vi "color image 2d.vi"(6 "path to JPEG file":path, 7 "Max":i32, 8 "Names":T2={"Red name"="Ca", "Green name"="Ca", "Blu name"="Ca"}, 9 "ROI-Blue":i32[][](graph), 10 "ROI-Green":i32[][](graph), 11 "ROI-Red":i32[][](graph)) -> ()   [LabVIEW 2023]
uses:
  <vilib>/Utility/miscctls.llb/LVBoundsTypeDef.ctl
  <vilib>/vision/Management.llb/Cast Image 2 Method.ctl
  <vilib>/vision/NI_Vision_Development_Module.lvlib
panel:
  out "Red":T1(plugin-control)
  out "Green":T1(plugin-control)
  out "Blue":T1(plugin-control)
  out "concatenated string":picture
  out "error out":errorcluster
  in  "error in":errorcluster
  out "Intensity Graph 6":u16[][](graph)
  out "Intensity Graph 5":u16[][](graph)
  out "Intensity Graph 4":u16[][](graph)
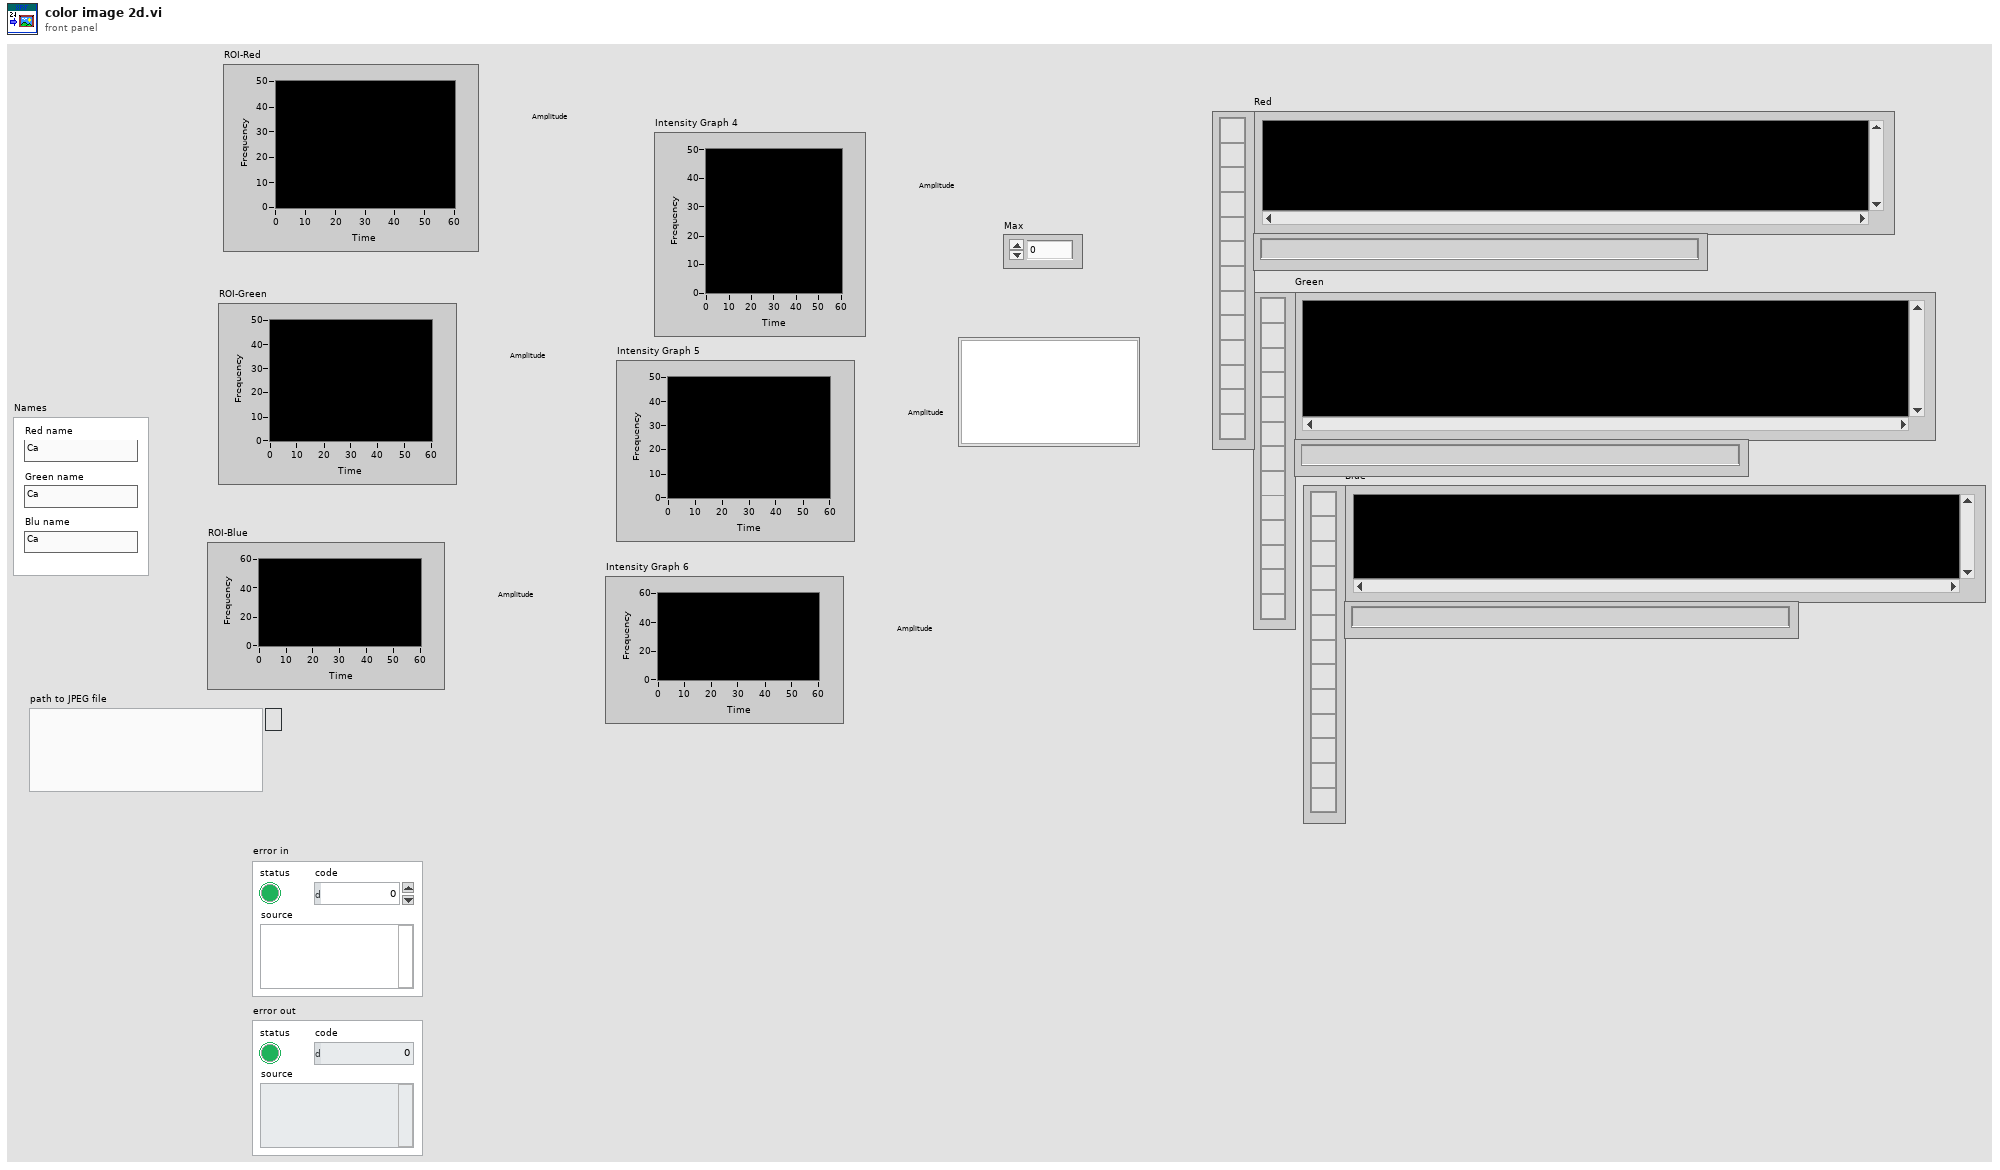
[diagram p1: front panel]
types:
  T1 = typedef "IMAQ Image.ctl" = refnum<image>
  T2 = cluster{"Red name":string, "Green name":string, "Blu name":string}
  T3 = typedef "Image Type" = u32
  T4 = typedef "Cast Image 2 Method.ctl" = u32
  T5 = typedef "LVBoundsTypeDef.ctl" = cluster{"Width":u32, "Height":u32}
  T6 = enum16{"User-specified Font", "Application Font", "System Font", "Dialog Font"}
  T7 = cluster{"Font Name:":string, "Size":i16, "Strikeout?":bool, "Italic?":bool, "Underline?":bool, "Outline?":bool, "Shadow?":bool, "Bold?":bool}
  T8 = typedef "imagedata.ctl" = cluster{"image type":i32, "image depth":i32, "image":u8[], "mask":u8[], "colors":u32[], "Rectangle":cluster{"left":i16, "top":i16, "right":i16, "bottom":i16}}
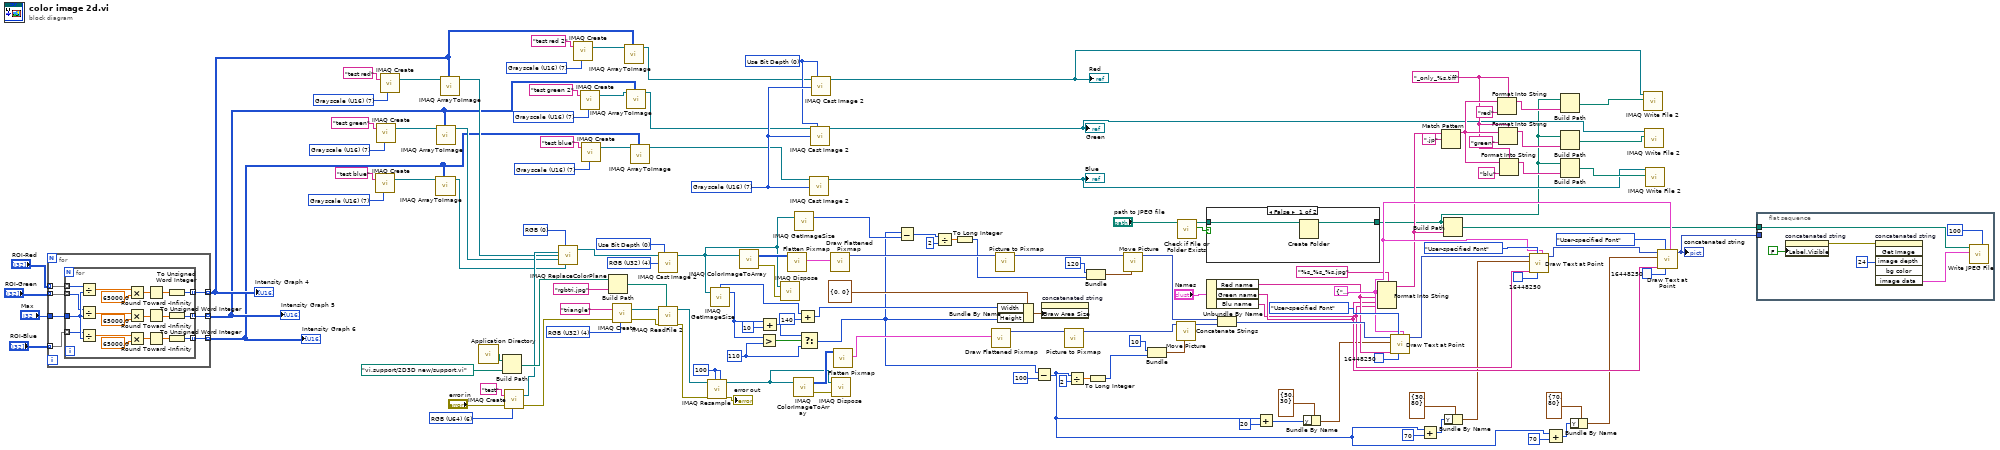
[diagram p0: block diagram]
diagram:
  w11 = T3 7 items=["Grayscale (U8)", "Grayscale (I16)", "Grayscale (SGL)", "Complex (CSG)", "RGB (U32)", "HSL (U32)", "RGB (U64)", "Grayscale (U16)"] ("Image Type")
  w13 = T3 7 items=["Grayscale (U8)", "Grayscale (I16)", "Grayscale (SGL)", "Complex (CSG)", "RGB (U32)", "HSL (U32)", "RGB (U64)", "Grayscale (U16)"] ("Image Type")
  w14 = T3 7 items=["Grayscale (U8)", "Grayscale (I16)", "Grayscale (SGL)", "Complex (CSG)", "RGB (U32)", "HSL (U32)", "RGB (U64)", "Grayscale (U16)"] ("Image Type")
  w17 = T4 0 items=["Use Bit Depth", "Shift", "Use Lookup Table"] ("Method")
  w18 = T3 7 items=["Grayscale (U8)", "Grayscale (I16)", "Grayscale (SGL)", "Complex (CSG)", "RGB (U32)", "HSL (U32)", "RGB (U64)", "Grayscale (U16)"] ("Image Type")
  w35 = "_only_%s.tiff" ("format string")
  w70 = u16 0 items=["RGB", "HSL", "HSV", "HSI"] ("Color Mode")
  w79 = T3 7 items=["Grayscale (U8)", "Grayscale (I16)", "Grayscale (SGL)", "Complex (CSG)", "RGB (U32)", "HSL (U32)", "RGB (U64)", "Grayscale (U16)"] ("Image Type")
  w76 = T3 7 items=["Grayscale (U8)", "Grayscale (I16)", "Grayscale (SGL)", "Complex (CSG)", "RGB (U32)", "HSL (U32)", "RGB (U64)", "Grayscale (U16)"] ("Image Type")
  w73 = T3 7 items=["Grayscale (U8)", "Grayscale (I16)", "Grayscale (SGL)", "Complex (CSG)", "RGB (U32)", "HSL (U32)", "RGB (U64)", "Grayscale (U16)"] ("Image Type")
  w84 = T3 4 items=["Grayscale (U8)", "Grayscale (I16)", "Grayscale (SGL)", "Complex (CSG)", "RGB (U32)", "HSL (U32)", "RGB (U64)", "Grayscale (U16)"] ("Image Type")
  w85 = T4 0 items=["Use Bit Depth", "Shift", "Use Lookup Table"] ("Method")
  w64 = u32 110 ("Height")
  w101 = T7 {"Font Name:"="Times", "Size"=18, "Strikeout?"=FALSE, "Italic?"=FALSE, "Underline?"=FALSE, "Outline?"=FALSE, "Shadow?"=FALSE, "Bold?"=TRUE} ("[user-specified font]")
  w125 = T3 4 items=["Grayscale (U8)", "Grayscale (I16)", "Grayscale (SGL)", "Complex (CSG)", "RGB (U32)", "HSL (U32)", "RGB (U64)", "Grayscale (U16)"] ("Image Type")
  w129 = 100
  w138 = T3 6 items=["Grayscale (U8)", "Grayscale (I16)", "Grayscale (SGL)", "Complex (CSG)", "RGB (U32)", "HSL (U32)", "RGB (U64)", "Grayscale (U16)"] ("Image Type")
  n1 = for {
    tunnel: "ROI-Red" -> [w150] mode=indexing
    tunnel: "ROI-Green" -> [w149] mode=indexing
    tunnel: "ROI-Blue" -> [w148] mode=indexing
    tunnel: "Max" -> [w147]
    tunnel: [w146] -> w6 mode=indexing
    tunnel: [w145] -> w5 mode=indexing
    tunnel: [w144] -> w4 mode=indexing
    n2 = for {
      tunnel: w150 -> [w169] mode=indexing
      tunnel: w149 -> [w159] mode=indexing
      tunnel: w148 -> [w160] mode=indexing
      tunnel: w147 -> [w161]
      tunnel: [w166] -> w146 mode=indexing
      tunnel: [w158] -> w145 mode=indexing
      tunnel: [w157] -> w144 mode=indexing
      n3 = Divide(x=w169, y=w161) -> (x/y=w154:dbl)
      n4 = Divide(x=w159, y=w161) -> (x/y=w155:dbl)
      n5 = Divide(x=w160, y=w161) -> (x/y=w156:dbl)
      n6 = Multiply(x=w154, y=65000.0) -> (x*y=w167:dbl)
      n7 = Multiply(x=w155, y=65000.0) -> (x*y=w165:dbl)
      n8 = Multiply(x=w156, y=65000.0) -> (x*y=w162:dbl)
      n9 = Round Toward -Infinity(1:w167) -> (0:w153:dbl)
      n10 = Round Toward -Infinity(1:w165) -> (0:w152:dbl)
      n11 = Round Toward -Infinity(1:w162) -> (0:w151:dbl)
      n12 = To Unsigned Word Integer(number=w153) -> (unsigned 16bit integer=w166:u16)
      n13 = To Unsigned Word Integer(number=w152) -> (unsigned 16bit integer=w158:u16)
      n14 = To Unsigned Word Integer(number=w151) -> (unsigned 16bit integer=w157:u16)
    }
  }
  "Intensity Graph 5" <- w5
  "Intensity Graph 6" <- w4
  "Intensity Graph 4" <- w6
  n15 = call "IMAQ Create"("Image Name"="test blue", "Image Type"=w79) -> ("New Image"=w80:T1)  [unwired: 3 in, 1 out]
  n16 = call "IMAQ Create"("Image Name"="test green", "Image Type"=w76) -> ("New Image"=w75:T1)  [unwired: 3 in, 1 out]
  n17 = call "IMAQ Create"("Image Name"="test red", "Image Type"=w73) -> ("New Image"=w74:T1)  [unwired: 3 in, 1 out]
  n18 = call "IMAQ ArrayToImage"("Image Pixels (U16)"=w4, "Image"=w80) -> ("Image Out"=w24:T1)  [unwired: 8 in, 1 out]
  n19 = call "IMAQ ArrayToImage"("Image Pixels (U16)"=w5, "Image"=w75) -> ("Image Out"=w22:T1)  [unwired: 8 in, 1 out]
  n20 = call "IMAQ ArrayToImage"("Image Pixels (U16)"=w6, "Image"=w74) -> ("Image Out"=w20:T1)  [unwired: 8 in, 1 out]
  n21 = call <vilib>:"Application Directory.vi"() -> ("Application Directory"=w131:path)
  n22 = Build Path(base path=w131, name or relative path=path "vi.support/2D3D new/support.vi") -> (appended path=w132:path)
  n23 = call "IMAQ Create"("Image Name"="test", "Image Type"=w138, "error in (no error)"="error in") -> ("New Image"=w69:T1, "error out"=w99:errorcluster)  [unwired: 2 in]
  n24 = call "IMAQ ReplaceColorPlane"("Color Mode"=w70, "Image Dst"=w69, "Red or Hue Plane"=w20, "Green or Sat Plane"=w22, "Blue or Luma or Val or Inten Plane"=w24) -> ("Image Dst Out"=w71:T1)  [unwired: 9 in, 1 out]
  n25 = call "IMAQ Create"("Image Name"="test red 2", "Image Type"=w14) -> ("New Image"=w8:T1)  [unwired: 3 in, 1 out]
  n26 = call "IMAQ Create"("Image Name"="test green 2", "Image Type"=w13) -> ("New Image"=w7:T1)  [unwired: 3 in, 1 out]
  n27 = call "IMAQ Create"("Image Name"="test blue", "Image Type"=w11) -> ("New Image"=w9:T1)  [unwired: 3 in, 1 out]
  n28 = Build Path(base path=w132, name or relative path="rgbtri.jpg") -> (appended path=w133:path)
  n29 = call "IMAQ Create"("Image Name"="triangle", "Image Type"=w125, "error in (no error)"=w99) -> ("New Image"=w136:T1, "error out"=w135:errorcluster)  [unwired: 2 in]
  n30 = call "IMAQ ArrayToImage"("Image Pixels (U16)"=w6, "Image"=w8) -> ("Image Out"=w3:T1)  [unwired: 8 in, 1 out]
  n31 = call "IMAQ ArrayToImage"("Image Pixels (U16)"=w5, "Image"=w7) -> ("Image Out"=w2:T1)  [unwired: 8 in, 1 out]
  n32 = call "IMAQ ArrayToImage"("Image Pixels (U16)"=w4, "Image"=w9) -> ("Image Out"=w1:T1)  [unwired: 8 in, 1 out]
  n33 = call "IMAQ Cast Image 2"("Image Src"=w71, "Method"=w85, "Image Type"=w84) -> ("Image Dst Out"=w63:T1)  [unwired: 11 in, 1 out]
  n34 = call "IMAQ ReadFile 2"("File Path"=w133, "error in (no error)"=w135, "Image"=w136) -> ("error out"=w126:errorcluster, "Image Out"=w128:T1)  [unwired: 4 in, 3 out]
  n35 = call "IMAQ Resample"("X Resolution"=w129, "Y Resolution"=w129, "error in (no error)"=w126, "Image Src"=w128) -> ("error out"=→"error out":errorcluster, "Image Dst Out"=w81:T1)  [unwired: 6 in]
  n36 = call "IMAQ GetImageSize"("Image"=w63) -> ("Y Resolution"=w67:i32, "X Resolution"=w96:i32)  [unwired: 3 in, 1 out]
  n37 = call "IMAQ ColorImageToArray"("Image"=w63) -> ("Image Pixels (U32)"=w124:u32[][], "error out"=w83:errorcluster)  [unwired: 3 in, 1 out]
  n38 = Greater?(x=w67, y=w64) -> (0:w68:bool)
  n39 = Add(x=w67, y=10) -> (x+y=w65:i32)
  n40 = call "IMAQ Dispose"("Image"=w63, "error in (no error)"=w83) -> ()  [unwired: 4 in, 1 out]
  n41 = call <vilib>:"Flatten Pixmap.vi"("24-bit pixmap"=w124) -> ("image data"=w123:T8)  [unwired: 10 in]
  n42 = call "IMAQ ColorImageToArray"("Image"=w81) -> ("Image Pixels (U32)"=w121:u32[][], "error out"=w82:errorcluster)  [unwired: 3 in, 1 out]
  n43 = call "IMAQ GetImageSize"("Image"=w63) -> ("Y Resolution"=w61:i32)  [unwired: 3 in, 2 out]
  n44 = Add(x=w96, y=140) -> (x+y=w62:i32)
  n45 = Select(t=w65, s=w68, f=w64) -> (s? t:f=w53:u32)
  n46 = call "IMAQ Cast Image 2"("Image Src"=w1, "Image Type"=w18) -> ("Image Dst Out"=w23:T1)  [unwired: 12 in, 1 out]
  "Blue" <- w23
  n47 = call "IMAQ Cast Image 2"("Image Src"=w2, "Method"=w17, "Image Type"=w18) -> ("Image Dst Out"=w21:T1)  [unwired: 11 in, 1 out]
  "Green" <- w21
  n48 = call "IMAQ Cast Image 2"("Image Src"=w3, "Method"=w17, "Image Type"=w18) -> ("Image Dst Out"=w19:T1)  [unwired: 11 in, 1 out]
  "Red" <- w19
  n49 = call <vilib>:"Draw Flattened Pixmap.vi"("image data"=w123) -> ("new picture"=w120:picture)  [unwired: 8 in]
  n50 = call "IMAQ Dispose"("Image"=w81, "error in (no error)"=w82) -> ()  [unwired: 4 in, 1 out]
  n51 = call <vilib>:"Flatten Pixmap.vi"("24-bit pixmap"=w121) -> ("image data"=w122:T8)  [unwired: 10 in]
  n52 = Subtract(x=w53, y=w61) -> (x-y=w57:u32)
  n53 = Divide(x=w57, y=2) -> (x/y=w59:dbl)
  n54 = To Long Integer(number=w59) -> (32bit integer=w58:i32)
  n55 = call <vilib>:"Draw Flattened Pixmap.vi"("image data"=w122) -> ("new picture"=w119:picture)  [unwired: 8 in]
  n56 = call <vilib>:"Picture to Pixmap.vi"("picture"=w120) -> ("new picture"=w115:picture)  [unwired: 9 in, 1 out]
  n57 = Bundle By Name(cluster=T5 {"Width"=0, "Height"=0} ("Draw Area Size"), "Width"=w62, "Height"=w53) -> (w97:T5)
  n58 = Subtract(x=w53, y=u32 100) -> (x-y=w39:u32)
  n59 = property on="concatenated string" class="Pict"("Draw Area Size"=w97) -> ()  [unwired: 2 in, 2 out]
  n60 = call <vilib>:"Picture to Pixmap.vi"("picture"=w119) -> ("new picture"=w118:picture)  [unwired: 9 in, 1 out]
  n61 = Divide(x=w39, y=2) -> (x/y=w56:dbl)
  n62 = Bundle(120, w58) -> (w114:cluster{i32, i32})  [unwired: 1 in]
  n63 = To Long Integer(number=w56) -> (32bit integer=w54:i32)
  n64 = call "Move Picture.vi"("Delta"=w114, "Picture In"=w115) -> ("value"=w112:picture)  [unwired: 8 in, 1 out]
  n65 = Bundle(10, w54) -> (w117:cluster{i32, i32})  [unwired: 1 in]
  n66 = call "Move Picture.vi"("Delta"=w117, "Picture In"=w118) -> ("value"=w116:picture)  [unwired: 8 in, 1 out]
  n67 = call <vilib>:"Check if File or Folder Exists.vi"("path"="path to JPEG file") -> ("file or folder exists?"=w92:bool, "dup path"=w91:path)  [unwired: 8 in, 1 out]
  n68 = case shown="False" w92 {
    tunnel: [w170 w172] -> w16
    tunnel: w91 -> [w171 w172]
    frame False {
      n69 = Create Folder(path (use dialog)=w171) -> (created path=w170:path)  [unwired: 2 in, 2 out]
    }
    frame True {
    }
  }
  n70 = Unbundle By Name("Names") -> ("Red name"=w89:string, "Green name"=w88:string, "Blu name"=w87:string)
  n71 = Concatenate Strings(w112, w116) -> (w110:picture)
  n72 = Add(x=w39, y=u32 20) -> (x+y=w49:u32)
  n73 = Bundle By Name(cluster=cluster{"x":i16, "y":i16} {"x"=50, "y"=30} ("origin"), "y"=w49) -> (w48:cluster{"x":i16, "y":i16})
  n74 = Format Into String(format string="%s_%s_%s.jpg", w89, w88, w87) -> (resulting string=w38:string)  [unwired: 2 in, 1 out]
  n75 = call <vilib>:"Draw Text at Point.vi"("[user-specified font]"=w101, "text color(black)"=u32 16448250, "desired font(Application)"=T6."User-specified Font", "text"=w89, "origin"=w48, "picture"=w110) -> ("new picture"=w103:picture)  [unwired: 4 in, 1 out]
  n76 = Add(x=w39, y=u32 70) -> (x+y=w44:u32)
  n77 = Match Pattern(string=w38, regular expression=".jp") -> (before substring=w36:string)  [unwired: 1 in, 3 out]
  n78 = Build Path(base path=w16, name or relative path=w38) -> (appended path=w28:path)
  n79 = Bundle By Name(cluster=cluster{"X":i32, "Y":i32} {"X"=30, "Y"=80} ("Origin"), "Y"=w44) -> (w46:cluster{"X":i32, "Y":i32})
  n80 = Format Into String(format string=w35, initial string=w36, "red" ("input 1")) -> (resulting string=w31:string)  [unwired: 1 in, 1 out]
  n81 = Format Into String(format string=w35, initial string=w36, "green" ("input 1")) -> (resulting string=w30:string)  [unwired: 1 in, 1 out]
  n82 = Format Into String(format string=w35, initial string=w36, "blu" ("input 1")) -> (resulting string=w29:string)  [unwired: 1 in, 1 out]
  n83 = call <vilib>:"Draw Text at Point.vi"("[user-specified font]"=w101, "text color(black)"=u32 16448250, "desired font(Application)"=T6."User-specified Font", "text"=w87, "origin"=w46, "picture"=w103) -> ("new picture"=w102:picture)  [unwired: 4 in, 1 out]
  n84 = Add(x=w39, y=u32 70) -> (x+y=w43:u32)
  n85 = Build Path(base path=w16, name or relative path=w29) -> (appended path=w25:path)
  n86 = Build Path(base path=w16, name or relative path=w31) -> (appended path=w27:path)
  n87 = Build Path(base path=w16, name or relative path=w30) -> (appended path=w26:path)
  n88 = Bundle By Name(cluster=cluster{"X":i32, "Y":i32} {"X"=70, "Y"=80} ("Origin"), "Y"=w43) -> (w40:cluster{"X":i32, "Y":i32})
  n89 = call-poly "IMAQ Write File 2"("File Path"=w27, "Image"=w19) -> ()  [unwired: 8 in, 2 out]
  n90 = call-poly "IMAQ Write File 2"("File Path"=w26, "Image"=w21) -> ()  [unwired: 8 in, 2 out]
  n91 = call-poly "IMAQ Write File 2"("File Path"=w25, "Image"=w23) -> ()  [unwired: 8 in, 2 out]
  n92 = call <vilib>:"Draw Text at Point.vi"("[user-specified font]"=w101, "text color(black)"=u32 16448250, "desired font(Application)"=T6."User-specified Font", "text"=w88, "origin"=w40, "picture"=w102) -> ("new picture"=w86:picture)  [unwired: 4 in, 1 out]
  "concatenated string" <- w86
  n93 = flat-sequence {
    tunnel: w86 -> [_]
    tunnel: w28 -> [w177]
    frame #0 {
      n94 = property on="concatenated string" class="Pict"("Label.Visible"=FALSE) -> (error out=w175:errorcluster)  [unwired: 2 in, 1 out]
      n95 = invoke on="concatenated string" class="Pict" method="Get Image"(error in=w175, "image depth"=24 ("Image Depth")) -> ("image data"=w178:T8)  [unwired: 4 in, 5 out]
      n96 = call <vilib>:"Write JPEG File.vi"("quality (80)"=100, "image data"=w178, "path to JPEG file"=w177) -> ()  [unwired: 7 in, 2 out]
    }
  }
